vi "Initialize (Remote Physical Channel).vi"(0 "physical channels":refnum<k21>, 1 "Hostname/IP":string, 2 "Port":u16, 3 "https?":bool, 7 "reservation access (Read/Write)":i32(ring)=3 items=["None"=0, "Read Only"=1, "Read/Write"=3], 9 "reservation group":string, 11 "error in (no error)":errorcluster, 12 "connect timeout (60 sec)":dbl=60.0, 13 "username":string="admin", 14 "password":string) -> (4 "SLSC Remote out":refnum<class "SLSC Remote.lvclass">, 15 "error out":errorcluster)   [LabVIEW 2015, in "SLSC Remote.lvclass"]
uses:
  SLSC Remote.lvclass
  SLSC Interface Class/slsc type.ctl
  SLSC Interface Class/SLSC Interface.lvclass
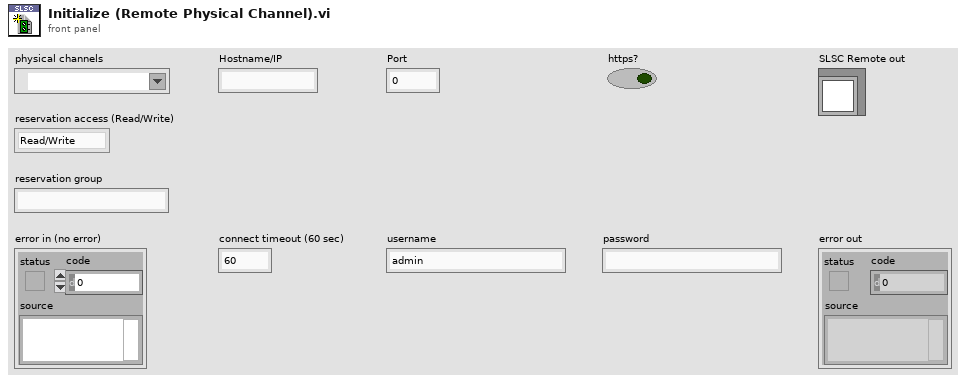
[diagram p1: front panel]
types:
  T1 = typedef "SLSC Interface.lvclass/slsc type.ctl" = enum16{"device", "nvmem", "channel", "none"}
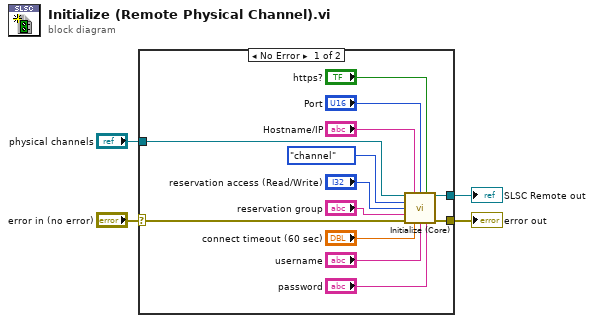
[diagram p0: block diagram]
diagram:
  n1 = case shown="No Error" "error in (no error)" {
    selector: "error in (no error)" -> [w16 w18]
    tunnel: [w14 w18] -> w3
    tunnel: [w15 _] -> w2
    tunnel: "physical channels" -> [w17 _]
    frame No Error {
      n2 = call "Initialize (Core).vi"("resources"=w17, "Hostname/IP"="Hostname/IP", "Port"="Port", "https?"="https?", "slsc type"=slsc_type."channel", "reservation access (Read/Write)"="reservation access (Read/Write)", "reservation group"="reservation group", "error in (no error)"=w16, "connect timeout (60 sec)"="connect timeout (60 sec)", "username"="username", "password"="password") -> ("SLSC Remote out"=w15:refnum<class "SLSC Remote.lvclass">, "error out"=w14:errorcluster)  [unwired: 3 in]
    }
    frame Error {
    }
  }
  "error out" <- w3
  "SLSC Remote out" <- w2
